vi "Target.vi"() -> ()   [LabVIEW 2018]
uses:
  <vilib>/Platform/TimedLoop/XDataNode/timing_clust.ctl
  <vilib>/Platform/TimedLoop/XDataNode/nitl_modes.ctl
  <vilib>/Platform/TimedLoop/XDataNode/wakeup.ctl
  <vilib>/rvi/eio/common/nirviEmuTemplateMethod_errors.vi
  <vilib>/rvi/Emulation/niFpgaGetClockAttributes.vi
  <vilib>/rvi/Emulation/niFpgaSctlEmulationGetInTimedLoop.vi
  <vilib>/rvi/Emulation/niFpgaEmulationReportErrorSimple.vi
  <vilib>/rvi/Emulation/niFpgaProcessEmulError.vi
  <vilib>/rvi/Emulation/niFpgaCriticalErrorInLSC.vi
  <vilib>/rvi/DataTransferAndStorage/Container/Common/niFpgaContainerGetUniqueNameForEmu.vi
  <vilib>/rvi/Memory/Memory_Emulation/niFpgaMemoryFastEmulationDramWriteAndRequestData.vi
  <vilib>/rvi/Memory/Memory_Emulation/niFpgaMemoryEmulationDramWriteAndRequestData.vi
  <vilib>/rvi/Memory/Memory_Emulation/niFpgaMemoryEmulationDramWriteAndRequestDataApplyByteEnables.vi
  <vilib>/rvi/interface/RandomDataEmulation/niFpgaRandomDataHandleErrors.vi
  <vilib>/eio/EIONode/EIONode.xnode
  <vilib>/Platform/TimedLoop/XDataNode/XDataNode.xnode
  <vilib>/rvi/DataTransferAndStorage/Container/XNode/niFpgaContainer.xnode
  <vilib>/rvi/Memory/Memory_Emulation/niFpgaMemoryEmulationDramRetrieveData.vi
  <vilib>/rvi/interface/RandomDataEmulation/nirviRandomDataFpgaReadWriteTemplate.vi
  <vilib>/Platform/TimedLoop/XDataNode/XDNodeRunTimeDep.lvlib
panel:
  in  "8_MISO":u8=8
  in  "18_OFF":u8=18
  in  "26_OFF":u8=26
  in  "18_MISO":u8=18
  in  "26_MISO":u8=26
  in  "18_CLK":u8=18
  in  "26_CLK":u8=26
  in  "15_MOSI":u8=15
  in  "23_MOSI":u8=23
  in  "R(T)/W(F)":bool
  in  "8(F)/16(T)":bool
  in  "Кадр в память":bool
  in  "1310720":u32=1310720
  in  "Направление бит":bool
  in  "Делитель (24/? = F, Гц)":u8=2
  in  "Стоп":bool
  out "SPI_OFF":bool
  in  "MOSI":bool[](array[boolean])=[FALSE, FALSE, FALSE, FALSE, FALSE, FALSE, FALSE, FALSE, FALSE, FALSE, FALSE, FALSE, FALSE, FALSE, FALSE, FALSE, FALSE, FALSE, FALSE, FALSE, FALSE, FALSE, FALSE, FALSE]
  out "MISO":bool[](array[boolean])
  in  "SPI":bool
  in  "RESET":bool
  in  "Автомат":bool
  out "Записали адресов":u32
  in  "Кадр на ПК":bool
  in  "Нач_адр":u32
  in  "Кон_адр":u32=163840
  out "Записали FIFO":bool
  in  "TRIG_1":u8=5
  in  "TRIG_2":u8=100
  in  "TRIG":bool
  # "FIFO 8 раз читается"
  # "0"
  # "0"
  # "1"
  # "1"
  # "2"
  # "2"
  # "3"
  # "3"
  # "4"
  # "4"
  # "5"
  # "5"
  # "6"
  # "6"
  # "7"
  # "При работе в 8-битном режиме MISO [7:0]"
  # "7"
  # "8"
  # "8"
  # "9"
  # "9"
  # "10"
  # "10"
  # "11"
  # "11"
  # "12"
  # "12"
  # "13"
  # "13"
  # "14"
  # "14"
  # "При работе в 8-битном режиме MOSI [15:8]"
  # "15"
  # "15"
  # "16"
  # "Тут адрес + R/W от HOST"
  # "17"
  # "18"
  # "19"
  # "20"
  # "21"
  # "22"
  # "23"
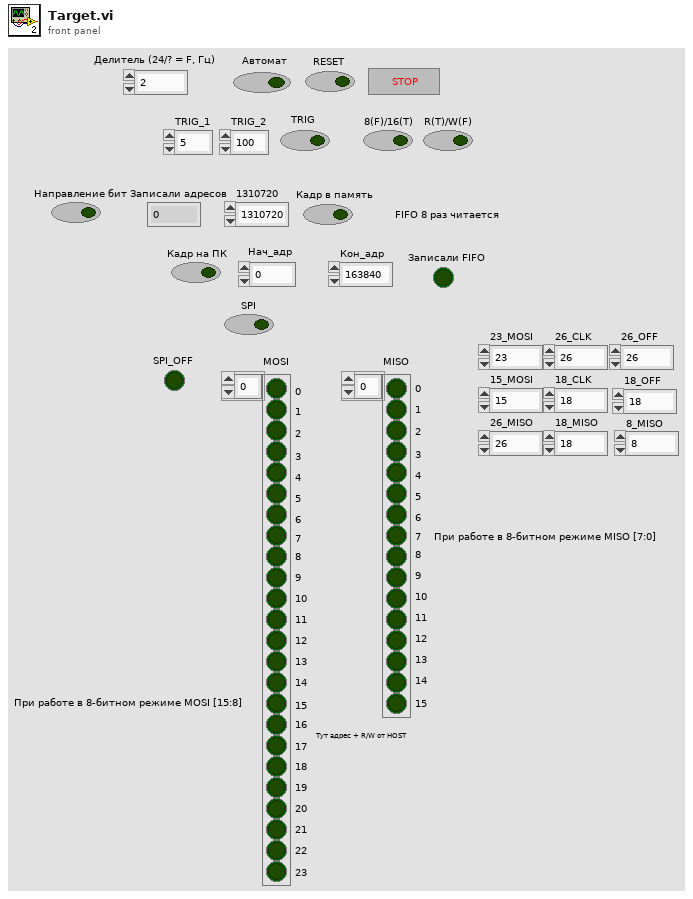
[diagram p1: front panel]
types:
  T1 = typedef "XDNodeRunTimeDep.lvlib/timing_clust.ctl" = cluster{"Expected End [f-1]":u64, "Actual End [f-1]":u64, "Finished Late? [f-1]":bool, "Expected End [i-1]":u64, "Actual End [i-1]":u64, "Finished Late? [i-1]":bool, "Expected Start [i]":u64, "Actual Start [i]":u64, "Expected Start [f]":u64, "Actual Start [f]":u64, "Source Name":string, "Structure Name":string, "Period":i64, "Deadline":i64, "Offset":i64, "Start":i64, "Priority":i32, "Timeout":i32, "Mode":T2, "Wakeup Reason":T3, "Error":errorcluster, "Source Type":string, "Secondary Source Type":string, "Global End Time":u64, "Global Start Time":u64, "Frame Duration":u64, "Iteration Duration":u64, "Assigned CPU":i32, "I/O Scan Engine Mode":u32}
  T2 = typedef "XDNodeRunTimeDep.lvlib/nitl_modes.ctl" = enum32{"No Change", "Process missed periods, maintain original phase", "Discard missed periods, maintain original phase", "Process missed periods, ignore original phase", "Discard missed periods, ignore original phase"}
  T3 = typedef "XDNodeRunTimeDep.lvlib/wakeup.ctl" = enum32{"Normal", "Aborted", "Asynchronous wakeup", "Timing source error", "Timed loop error", "Timeout"}
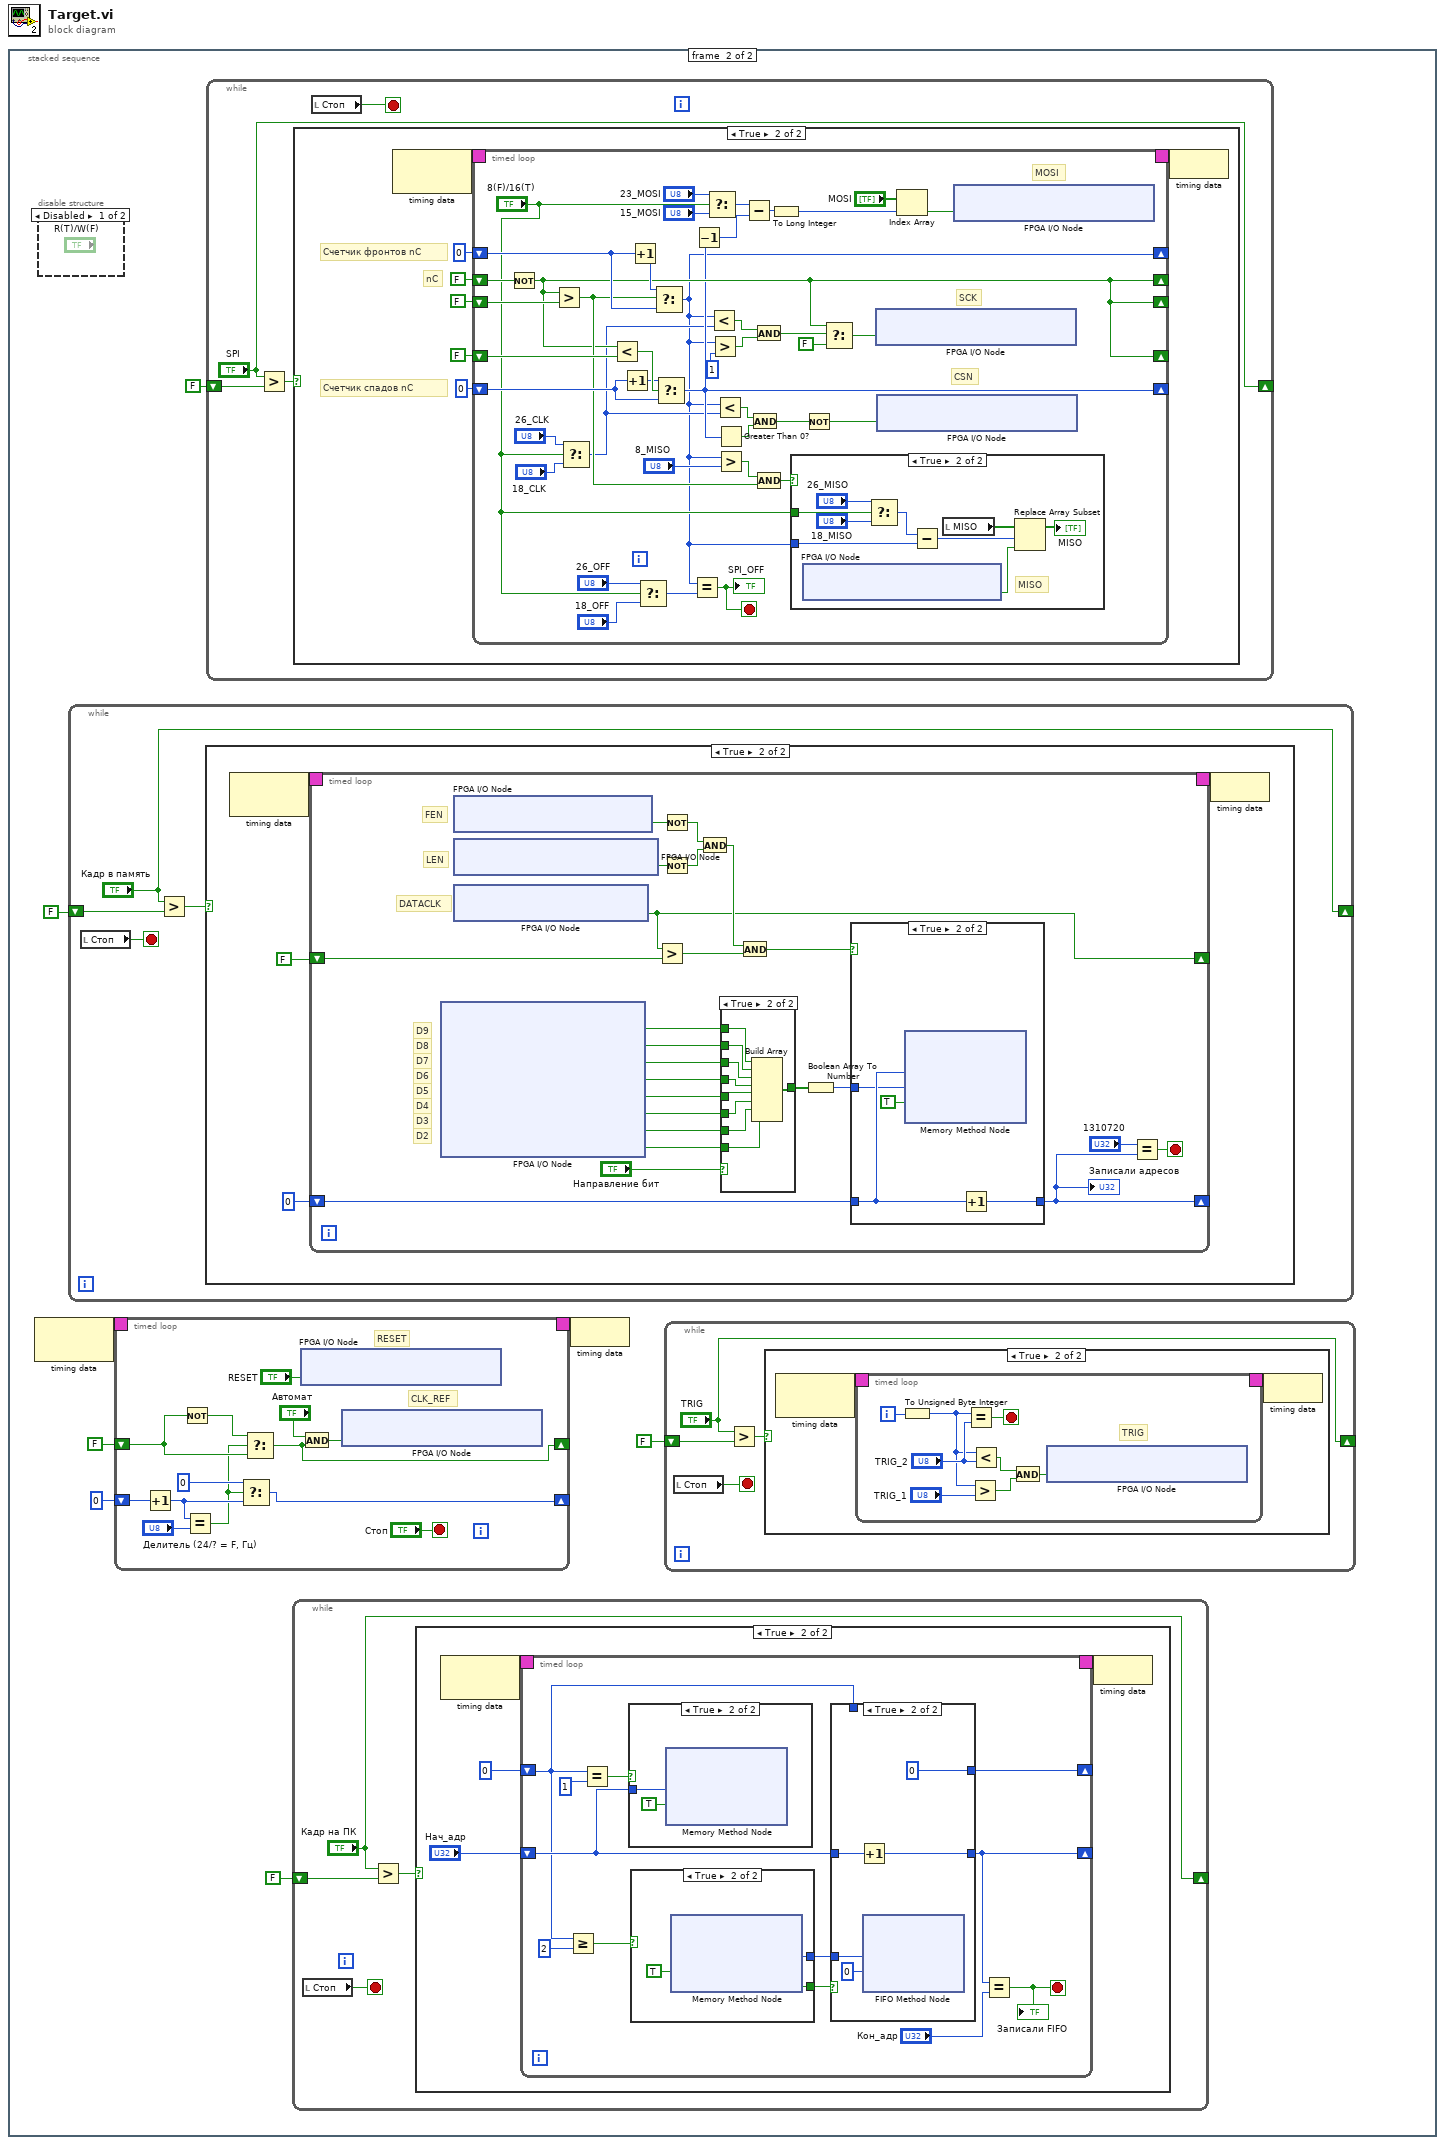
[diagram p0: block diagram]
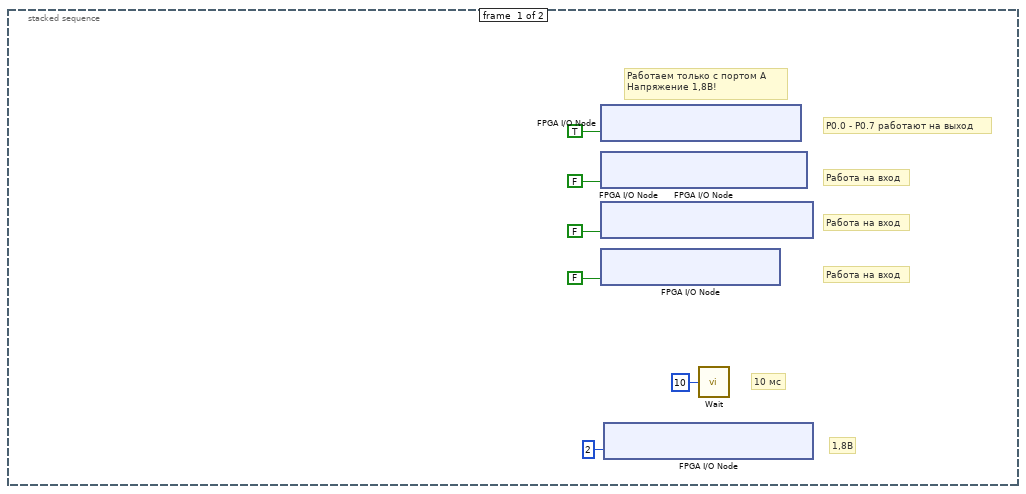
[diagram p2: hidden frame]
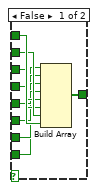
[diagram p5: hidden frame]
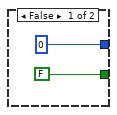
[diagram p9: hidden frame]
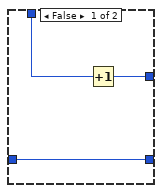
[diagram p11: hidden frame]
diagram:
  n1 = stacked-sequence {
    frame #0 {
      # "10 мс"
      # "1,8В"
      # "Работа на вход"
      # "Работа на вход"
      # "Работа на вход"
      # "P0.0 - P0.7 работают на выход"
      # "Работаем только с портом A\nНапряжение 1,8В!"
      n2 = xnode "FPGA I/O Node"("IO Module\\DDCA_DIO0-7_WE"=TRUE ("IO Module\\DDCA_DIO0-7_WE")) -> ()  [unwired: 1 in, 1 out]
      n3 = xnode "FPGA I/O Node"("IO Module\\DDCA_DIO8-15_WE"=FALSE ("IO Module\\DDCA_DIO8-15_WE")) -> ()  [unwired: 1 in, 1 out]
      n4 = xnode "FPGA I/O Node"("IO Module\\DDCA_DIO16-23_WE"=FALSE ("IO Module\\DDCA_DIO16-23_WE")) -> ()  [unwired: 1 in, 1 out]
      n5 = xnode "FPGA I/O Node"("IO Module\\DDCA_PFI_WE"=FALSE ("IO Module\\DDCA_DIO16-23_WE")) -> ()  [unwired: 1 in, 1 out]
      n6 = xnode "FPGA I/O Node"("IO Module\\Local_Supply_Select"=u8 2 ("IO Module\\Local_Supply_Select")) -> ()  [unwired: 1 in, 1 out]
      n7 = call "Wait"("Count(mSec)"=u8 10 ("Count(uSec)")) -> ()  [unwired: 1 out]
    }
    frame #1 {
      n8 = node-c288() -> (w12:T1)  [unwired: 1 in]
      n9 = disable-structure shown="Disabled" {
        frame Disabled {
        }
        frame Enabled {
        }
      }
      n10 = while {
        shift-right: ["Кадр в память"] -> _
        shift-left: FALSE -> [w17]
        stop <- w18 stop-if-true
        n11 = local read "Стоп"() -> (w18:bool)
        n12 = Greater?(x="Кадр в память", y=w17) -> (0:w16:bool)
        n13 = case shown="True" w16 {
          frame False {
          }
          frame True {
            n14 = node-c288() -> (w22:T1)  [unwired: 1 in]
            n15 = timed-loop {
              timing: w22 -> [_]
              timing-out: [_] -> w21
              shift-right: [w39] -> _
              shift-left: FALSE -> [w42]
              shift-right: [w25] -> _
              shift-left: u32 0 -> [w37]
              stop <- w23 stop-if-true
              # "DATACLK"
              # "D2"
              # "D3"
              # "D4"
              # "D5"
              # "D6"
              # "D7"
              # "D8"
              # "D9"
              # "LEN"
              # "FEN"
              n16 = xnode "FPGA I/O Node"() -> ("IO Module\\DDCA_DIO11_Read"=w35:bool, "IO Module\\DDCA_DIO12_Read"=w34:bool, "IO Module\\DDCA_DIO13_Read"=w33:bool, "IO Module\\DDCA_DIO14_Read"=w32:bool, "IO Module\\DDCA_DIO15_Read"=w31:bool, "IO Module\\DDCA_DIO16_Read"=w30:bool, "IO Module\\DDCA_DIO18_Read"=w29:bool, "IO Module\\DDCA_DIO17_Read"=w28:bool)  [unwired: 8 in, 8 out]
              n17 = xnode "FPGA I/O Node"() -> ("IO Module\\DDCA_DIO9_Read"=w46:bool)  [unwired: 1 in, 1 out]
              n18 = xnode "FPGA I/O Node"() -> ("IO Module\\DDCA_DIO10_Read"=w45:bool)  [unwired: 1 in, 1 out]
              n19 = xnode "FPGA I/O Node"() -> ("IO Module\\DDCA_PFI2_Read"=w39:bool)  [unwired: 1 in, 1 out]
              n20 = Greater?(x=w39, y=w42) -> (0:w40:bool)
              n21 = Not(x=w46) -> (.not. x?=w44:bool)
              n22 = Not(x=w45) -> (.not. x?=w43:bool)
              n23 = And(x=w44, y=w43) -> (x .and. y?=w41:bool)
              n24 = case shown="True" "Направление бит" {
                tunnel: w35 -> [w54 w64]
                tunnel: w34 -> [w53 w63]
                tunnel: w33 -> [w52 w62]
                tunnel: w32 -> [w51 w61]
                tunnel: w31 -> [w50 w60]
                tunnel: w30 -> [w49 w59]
                tunnel: w29 -> [w48 w58]
                tunnel: w28 -> [w47 w57]
                tunnel: [w55 w56] -> w27
                frame False {
                  n25 = Build Array(w47, w48, w49, w50, w51, w52, w53, w54) -> (w55:bool[])
                }
                frame True {
                  n26 = Build Array(w64, w63, w62, w61, w60, w59, w58, w57) -> (w56:bool[])
                }
              }
              n27 = And(x=w41, y=w40) -> (x .and. y?=w38:bool)
              n28 = Boolean Array To Number(Boolean array=w27) -> (number=w26:u8)
              n29 = case shown="True" w38 {
                tunnel: w37 -> [w65 w69]
                tunnel: [w65 w68] -> w25
                tunnel: w26 -> [_ w67]
                frame False {
                }
                frame True {
                  n30 = xnode ("Memory Method Node")("Address"=w69, "Data"=w67, "Input Valid"=TRUE) -> ()  [unwired: 1 in, 2 out]
                  n31 = Increment(x=w69) -> (x+1=w68:u32)
                }
              }
              "Записали адресов" <- w25
              n32 = Equal?(x="1310720", y=w25) -> (x = y?=w23:bool)
            }
            n33 = node-c288(w21) -> ()
          }
        }
      }
      n34 = timed-loop {
        timing: w12 -> [_]
        timing-out: [_] -> w11
        shift-right: [w93] -> _
        shift-left: FALSE -> [w96]
        shift-right: [w98] -> _
        shift-left: u8 0 -> [w102]
        stop <- "Стоп" stop-if-true
        # "RESET"
        # "CLK_REF"
        n35 = Increment(x=w102) -> (x+1=w100:u8)
        n36 = Not(x=w96) -> (.not. x?=w97:bool)
        n37 = Equal?(x=w100, y="Делитель (24/? = F, Гц)") -> (x = y?=w95:bool)
        n38 = Select(t=u8 0, s=w95, f=w100) -> (s? t:f=w98:u8)
        n39 = Select(t=w97, s=w95, f=w96) -> (s? t:f=w93:bool)
        n40 = xnode "FPGA I/O Node"("IO Module\\DDCA_DIO2_Write"="RESET") -> ()  [unwired: 1 in, 1 out]
        n41 = And(x="Автомат", y=w93) -> (x .and. y?=w104:bool)
        n42 = xnode "FPGA I/O Node"("IO Module\\DDCA_DIO1_Write"=w104) -> ()  [unwired: 1 in, 1 out]
      }
      n43 = while {
        shift-right: ["SPI"] -> _
        shift-left: FALSE ("SPI") -> [w150]
        stop <- w148 stop-if-true
        n44 = Greater?(x="SPI", y=w150) -> (0:w151:bool)
        n45 = case shown="True" w151 {
          frame False {
          }
          frame True {
            # "Счетчик фронтов nC"
            # "Счетчик спадов nC"
            # "nC"
            n46 = node-c288() -> (w158:T1)  [unwired: 1 in]
            n47 = timed-loop {
              timing: w158 -> [_]
              timing-out: [_] -> w157
              shift-right: [w184] -> _
              shift-left: FALSE -> [w199]
              shift-right: [w184] -> _
              shift-left: FALSE -> [w198]
              shift-right: [w159] -> _
              shift-left: u8 0 -> [w197]
              shift-right: [w184] -> _
              shift-left: FALSE -> [w196]
              shift-right: [w169] -> _
              shift-left: u8 0 -> [w193]
              stop <- w161 stop-if-true
              # "MOSI"
              # "CSN"
              # "SCK"
              n48 = Not(x=w199) -> (.not. x?=w184:bool)
              n49 = Greater?(x=w184, y=w198) -> (0:w185:bool)
              n50 = Select(t="26_CLK", s="8(F)/16(T)", f="18_CLK") -> (s? t:f=w162:u8)
              n51 = Less?(x=w184, y=w196) -> (x < y?=w195:bool)
              n52 = Increment(x=w193) -> (x+1=w194:u8)
              n53 = Increment(x=w197) -> (x+1=w188:u8)
              n54 = Select(t="26_OFF", s="8(F)/16(T)", f="18_OFF") -> (s? t:f=w165:u8)
              n55 = Select(t=w188, s=w185, f=w197) -> (s? t:f=w159:u8)
              n56 = Select(t=w194, s=w195, f=w193) -> (s? t:f=w169:u8)
              n57 = Equal?(x=w159, y=w165) -> (x = y?=w161:bool)
              "SPI_OFF" <- w161
              n58 = Decrement(x=w169) -> (x-1=w177:u8)
              n59 = Select(t="23_MOSI", s="8(F)/16(T)", f="15_MOSI") -> (s? t:f=w174:u8)
              n60 = Less?(x=w159, y=w162) -> (x < y?=w183:bool)
              n61 = Greater?(x=w159, y=u8 1 ("1")) -> (0:w182:bool)
              n62 = Less?(x=w159, y=w162) -> (x < y?=w189:bool)
              n63 = Greater Than 0?(x=w169) -> (x > 0?=w190:bool)
              n64 = Greater?(x=w159, y="8_MISO") -> (0:w186:bool)
              n65 = Subtract(x=w174, y=w177) -> (x-y=w171:u8)
              n66 = And(x=w189, y=w190) -> (x .and. y?=w181:bool)
              n67 = And(x=w183, y=w182) -> (x .and. y?=w191:bool)
              n68 = Compound Arithmetic op=AND(w186, w185) -> (w187:bool)
              n69 = To Long Integer(number=w171) -> (32bit integer=w170:i32)
              n70 = case shown="True" w187 {
                tunnel: w159 -> [_ w205]
                tunnel: "8(F)/16(T)" -> [_ w201]
                frame False {
                }
                frame True {
                  # "MISO"
                  n71 = xnode "FPGA I/O Node"() -> ("IO Module\\DDCA_DIO8_Read"=w206:bool)  [unwired: 1 in, 1 out]
                  n72 = Select(t="26_MISO", s=w201, f="18_MISO") -> (s? t:f=w202:u8)
                  n73 = Subtract(x=w202, y=w205) -> (x-y=w204:u8)
                  n74 = local read "MISO"() -> (w207:bool[])
                  n75 = Replace Array Subset(array=w207, new element=w206, index=w204) -> (→"MISO":bool[])
                }
              }
              n76 = Not(x=w181) -> (.not. x?=w178:bool)
              n77 = Select(t=w184, s=w191, f=FALSE) -> (s? t:f=w179:bool)
              n78 = xnode "FPGA I/O Node"("IO Module\\DDCA_DIO6_Write"=w179) -> ()  [unwired: 1 in, 1 out]
              n79 = xnode "FPGA I/O Node"("IO Module\\DDCA_DIO4_Write"=w178) -> ()  [unwired: 1 in, 1 out]
              n80 = Index Array(array="MOSI", index=w170) -> (element=w180:bool)
              n81 = xnode "FPGA I/O Node"("IO Module\\DDCA_DIO5_Write"=w180) -> ()  [unwired: 1 in, 1 out]
            }
            n82 = node-c288(w157) -> ()
          }
        }
        n83 = local read "Стоп"() -> (w148:bool)
      }
      n84 = while {
        shift-right: ["Кадр на ПК"] -> _
        shift-left: FALSE ("Кадр на ПК") -> [w110]
        stop <- w112 stop-if-true
        n85 = local read "Стоп"() -> (w112:bool)
        n86 = Greater?(x="Кадр на ПК", y=w110) -> (0:w111:bool)
        n87 = case shown="True" w111 {
          frame False {
          }
          frame True {
            n88 = node-c288() -> (w116:T1)  [unwired: 1 in]
            n89 = timed-loop {
              shift-right: [w127] -> _
              shift-left: "Нач_адр" -> [w121]
              timing: w116 -> [_]
              timing-out: [_] -> w115
              shift-right: [w118] -> _
              shift-left: u8 0 -> [w119]
              stop <- w128 stop-if-true
              n90 = Greater Or Equal?(x=w119, y=u8 2 ("2")) -> (x >= y?=w122:bool)
              n91 = Equal?(x=w119, y=u8 1 ("1")) -> (x = y?=w125:bool)
              n92 = case shown="True" w125 {
                tunnel: w121 -> [_ w134]
                frame False {
                }
                frame True {
                  n93 = xnode ("Memory Method Node")("Address"=w134, "Input Valid"=TRUE) -> ()  [unwired: 1 in, 2 out]
                }
              }
              n94 = case shown="True" w122 {
                tunnel: [u8 0 ("Data") w132] -> w126
                tunnel: [FALSE ("Output Valid") w131] -> w120
                frame False {
                }
                frame True {
                  n95 = xnode ("Memory Method Node")("Ready for Output"=TRUE ("Ready For Output")) -> ("Data"=w132:u8, "Output Valid"=w131:bool)  [unwired: 1 in, 1 out]
                }
              }
              n96 = case shown="True" w120 {
                tunnel: [w136 w143] -> w127
                tunnel: w126 -> [_ w139]
                tunnel: w121 -> [w136 w142]
                tunnel: w119 -> [w138 _]
                tunnel: [w137 u8 0] -> w118
                frame False {
                  n97 = Increment(x=w138) -> (x+1=w137:u8)
                }
                frame True {
                  n98 = Increment(x=w142) -> (x+1=w143:u32)
                  n99 = xnode ("FIFO Method Node")("Element"=w139, "Timeout"=0) -> ()  [unwired: 1 in, 2 out]
                }
              }
              n100 = Equal?(x=w127, y="Кон_адр") -> (x = y?=w128:bool)
              "Записали FIFO" <- w128
            }
            n101 = node-c288(w115) -> ()
          }
        }
      }
      n102 = node-c288(w11) -> ()
      n103 = while {
        shift-right: ["TRIG"] -> _
        shift-left: FALSE ("TRIG") -> [w76]
        stop <- w74 stop-if-true
        n104 = local read "Стоп"() -> (w74:bool)
        n105 = Greater?(x="TRIG", y=w76) -> (0:w77:bool)
        n106 = case shown="True" w77 {
          frame False {
          }
          frame True {
            n107 = node-c288() -> (w79:T1)  [unwired: 1 in]
            n108 = timed-loop {
              timing: w79 -> [_]
              timing-out: [_] -> w78
              i -> [w81]
              stop <- w84 stop-if-true
              # "TRIG"
              n109 = To Unsigned Byte Integer(number=w81) -> (unsigned 8bit integer=w80:u8)
              n110 = Equal?(x=w80, y="TRIG_2") -> (x = y?=w84:bool)
              n111 = Greater?(x=w80, y="TRIG_1") -> (0:w86:bool)
              n112 = Less?(x=w80, y="TRIG_2") -> (x < y?=w87:bool)
              n113 = And(x=w87, y=w86) -> (x .and. y?=w83:bool)
              n114 = xnode "FPGA I/O Node"("IO Module\\DDCA_DIO3_Write"=w83) -> ()  [unwired: 1 in, 1 out]
            }
            n115 = node-c288(w78) -> ()
          }
        }
      }
    }
  }
